vi "VD2_TRABS_Calc.vi"(8 "error in (no error)":errorcluster, 10 "Exp name":string, 11 "Control-Client in":refnum<class "Control-Client.lvclass">) -> (0 "error out":errorcluster, 3 "Control-Client out":refnum<class "Control-Client.lvclass">)   [LabVIEW 2018, in "Control-Client.lvclass"]
uses:
  Control-Client.lvclass
  Experiments/Experiment.lvclass
  Control-Client.lvclass/Control-Client.ctl
  methods/Read Group #.vi
  Experiments/Experiments_group.lvclass
panel:
  out "Item Names":string[](array[string])
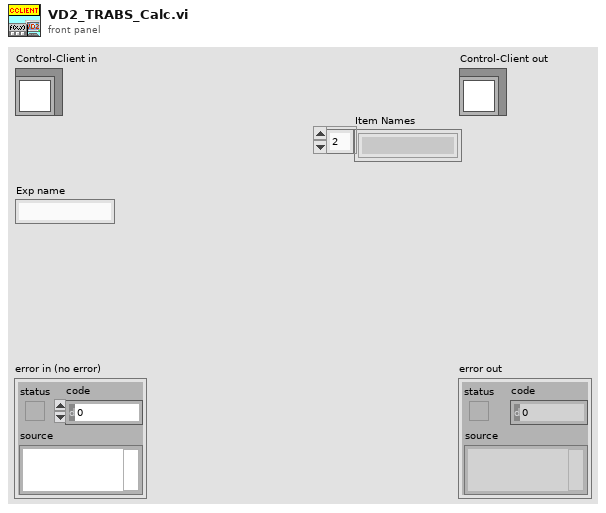
[diagram p1: front panel]
types:
  T1 = typedef "mylistbox.ctl" = i32[]
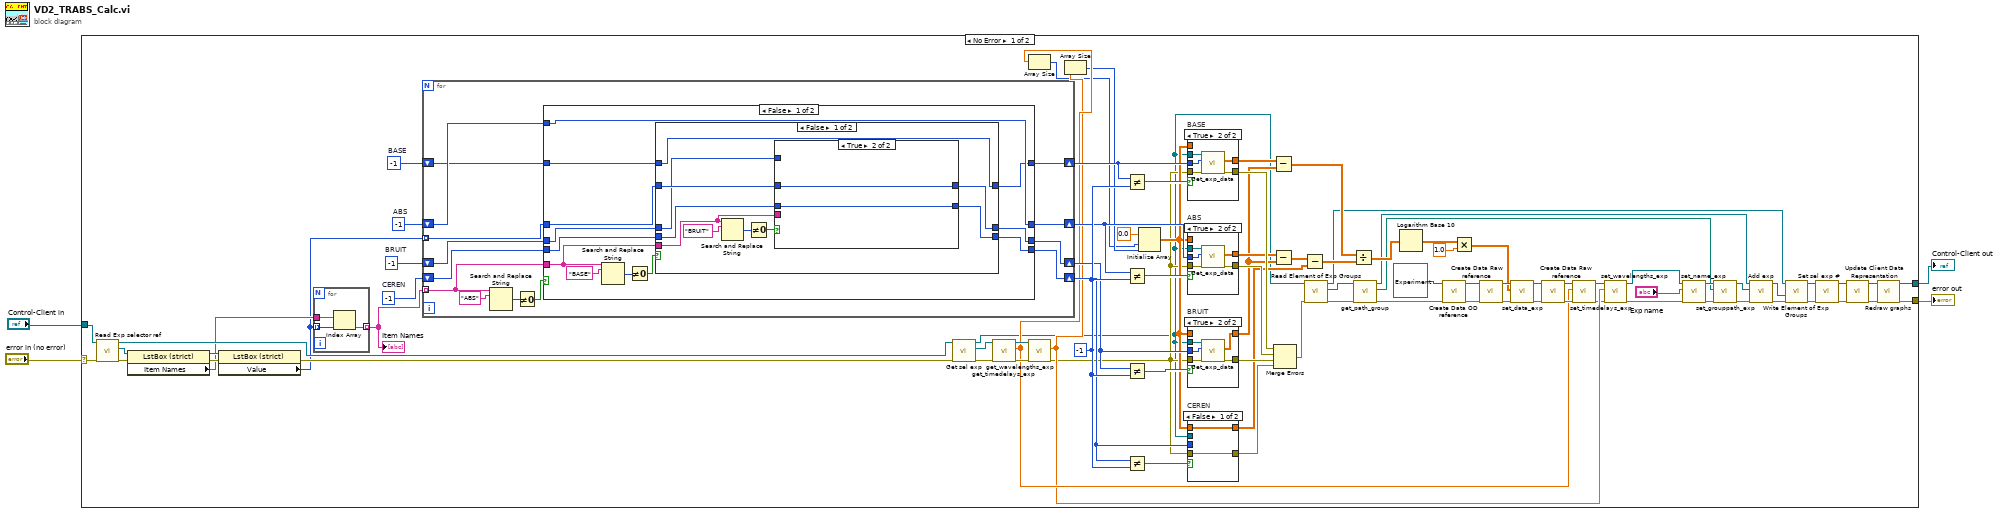
[diagram p0: block diagram]
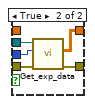
[diagram p2: hidden frame]
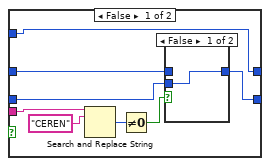
[diagram p6: hidden frame]
diagram:
  n1 = case shown="No Error" "error in (no error)" {
    selector: "error in (no error)" -> [w89 w177]
    tunnel: [w30 w177] -> w3
    tunnel: [w29 w176] -> w1
    tunnel: "Control-Client in" -> [w90 w176]
    frame No Error {
      w79 = -1 ("y")
      w85 = -1  # CEREN
      w84 = -1  # BRUIT
      w83 = -1  # BASE
      w82 = -1  # ABS
      n2 = call "Read Exp selector ref.vi"("error in (no error)"=w89, "Control-Client in"=w90) -> ("error out"=w88:errorcluster, "Exp selector ref"=w87:refnum<vi>, "Control-Client out"=w68:refnum<class "Control-Client.lvclass">)  [unwired: 7 in]
      n3 = property on="Property Node" class="LstBox (strict)"(reference=w87, error in=w88) -> (reference out=w86:refnum<vi>, error out=w19:errorcluster, "Item Names"=w17:string[])
      n4 = property class="LstBox (strict)"(reference=w86, error in=w19) -> (error out=w20:errorcluster, "Value"=w15:T1)  [unwired: 1 out]
      n5 = for {
        tunnel: w15 -> [w92] mode=indexing
        tunnel: w17 -> [w93]
        tunnel: [w91] -> w16 mode=indexing
        n6 = Index Array(array=w93, index=w92) -> (element=w91:string)
      }
      "Item Names" <- w16
      n7 = for {
        tunnel: w16 -> [w129] mode=indexing
        shift-right: [w124] -> w70
        shift-left: w85 -> [w123]
        shift-right: [w126] -> w69
        shift-left: w84 -> [w125]
        shift-right: [w128] -> w72
        shift-left: w83 -> [w127]
        shift-right: [w131] -> w71
        shift-left: w82 -> [w130]
        tunnel: w15 -> [w122] mode=indexing
        n8 = Search and Replace String(input string=w129, search string="ABS") -> (number of replacements=w133:i32)  [unwired: 6 in, 3 out]
        n9 = Not Equal To 0?(x=w133) -> (x != 0?=w132:bool)
        n10 = case shown="False" w132 {
          tunnel: [w146 w175] -> w131
          tunnel: w122 -> [w141 w175]
          tunnel: w130 -> [w146 _]
          tunnel: w129 -> [w139 _]
          tunnel: [w142 w174] -> w128
          tunnel: w127 -> [w140 w174]
          tunnel: [w138 w173] -> w126
          tunnel: w125 -> [w137 w173]
          tunnel: [w136 w172] -> w124
          tunnel: w123 -> [w135 w172]
          frame False {
            n11 = Search and Replace String(input string=w139, search string="BASE") -> (number of replacements=w144:i32)  [unwired: 6 in, 3 out]
            n12 = Not Equal To 0?(x=w144) -> (x != 0?=w143:bool)
            n13 = case shown="False" w143 {
              tunnel: [w156 w171] -> w142
              tunnel: w141 -> [w151 w171]
              tunnel: w140 -> [w156 _]
              tunnel: w139 -> [w149 _]
              tunnel: [w152 w170] -> w138
              tunnel: w137 -> [w150 w170]
              tunnel: [w148 w169] -> w136
              tunnel: w135 -> [w147 w169]
              frame False {
                n14 = Search and Replace String(input string=w149, search string="BRUIT") -> (number of replacements=w154:i32)  [unwired: 6 in, 3 out]
                n15 = Not Equal To 0?(x=w154) -> (x != 0?=w153:bool)
                n16 = case shown="True" w153 {
                  tunnel: [w164 w168] -> w152
                  tunnel: w151 -> [w158 w168]
                  tunnel: w150 -> [w164 _]
                  tunnel: w149 -> [w160 _]
                  tunnel: [w159 w167] -> w148
                  tunnel: w147 -> [w157 w167]
                  frame False {
                    n17 = Search and Replace String(input string=w160, search string="CEREN") -> (number of replacements=w162:i32)  [unwired: 6 in, 3 out]
                    n18 = Not Equal To 0?(x=w162) -> (x != 0?=w161:bool)
                    n19 = case shown="False" w161 {
                      tunnel: [w165 w166] -> w159
                      tunnel: w158 -> [_ w166]
                      tunnel: w157 -> [w165 _]
                      frame False {
                      }
                      frame True {
                      }
                    }
                  }
                  frame True {
                  }
                }
              }
              frame True {
              }
            }
          }
          frame True {
          }
        }
      }
      n20 = call "Get sel exp.vi"("error in (no error)"=w20, "Control-Client in"=w68) -> ("error out"=w66:errorcluster, "Sel experiment"=w65:refnum<class "Experiment.lvclass">, "Control-Client out"=w7:refnum<class "Control-Client.lvclass">)  [unwired: 7 in]
      n21 = call "get_timedelays_exp.vi"("error in (no error)"=w66, "Experiment.lvclass in"=w65) -> ("error out"=w67:errorcluster, "timedelays"=w27:dbl[], "Experiment.lvclass out"=w64:refnum<class "Experiment.lvclass">)  [unwired: 7 in]
      n22 = Array Size(array=w27) -> (size(s)=w5:i32)
      n23 = call "get_wavelengths_exp.vi"("error in (no error)"=w67, "Experiment.lvclass in"=w64) -> ("error out"=w18:errorcluster, "wavelengths"=w25:dbl[])  [unwired: 7 in, 1 out]
      n24 = Array Size(array=w25) -> (size(s)=w6:i32)
      n25 = Not Equal?(x=w72, y=w79) -> (x != y?=w81:bool)
      n26 = Not Equal?(x=w71, y=w79) -> (x != y?=w80:bool)
      n27 = Not Equal?(x=w69, y=w79) -> (x != y?=w78:bool)
      n28 = Not Equal?(x=w70, y=w79) -> (x != y?=w77:bool)
      n29 = Initialize Array(0.0 ("element"), w5, w6) -> (w62:dbl[][])
      n30 = case "BASE" shown="True" w81 {
        tunnel: w18 -> [w115 w121]
        tunnel: [w115 w120] -> w76
        tunnel: w7 -> [_ w119]
        tunnel: w72 -> [_ w117]
        tunnel: [w116 w118] -> w61
        tunnel: w62 -> [w116 _]
        frame False {
        }
        frame True {
          n31 = call "Get_exp_data.vi"("error in (no error)"=w121, "index"=w117, "Control-Client in"=w119) -> ("error out"=w120:errorcluster, "Data"=w118:sgl[][])  [unwired: 6 in, 1 out]
        }
      }
      n32 = case "ABS" shown="True" w80 {
        tunnel: w18 -> [w108 w114]
        tunnel: [w108 w113] -> w75
        tunnel: w7 -> [_ w112]
        tunnel: w71 -> [_ w110]
        tunnel: [w109 w111] -> w60
        tunnel: w62 -> [w109 _]
        frame False {
        }
        frame True {
          n33 = call "Get_exp_data.vi"("error in (no error)"=w114, "index"=w110, "Control-Client in"=w112) -> ("error out"=w113:errorcluster, "Data"=w111:sgl[][])  [unwired: 6 in, 1 out]
        }
      }
      n34 = case "BRUIT" shown="True" w78 {
        tunnel: w18 -> [w101 w107]
        tunnel: [w101 w106] -> w74
        tunnel: w7 -> [_ w105]
        tunnel: w69 -> [_ w103]
        tunnel: [w102 w104] -> w59
        tunnel: w62 -> [w102 _]
        frame False {
        }
        frame True {
          n35 = call "Get_exp_data.vi"("error in (no error)"=w107, "index"=w103, "Control-Client in"=w105) -> ("error out"=w106:errorcluster, "Data"=w104:sgl[][])  [unwired: 6 in, 1 out]
        }
      }
      n36 = case "CEREN" shown="False" w77 {
        tunnel: w18 -> [w95 w100]
        tunnel: [w95 w99] -> w73
        tunnel: w7 -> [_ w98]
        tunnel: w70 -> [_ w96]
        tunnel: [w94 w97] -> w57
        tunnel: w62 -> [w94 _]
        frame False {
        }
        frame True {
          n37 = call "Get_exp_data.vi"("error in (no error)"=w100, "index"=w96, "Control-Client in"=w98) -> ("error out"=w99:errorcluster, "Data"=w97:sgl[][])  [unwired: 6 in, 1 out]
        }
      }
      n38 = Subtract(x=w61, y=w59) -> (x-y=w55:dbl[][])
      n39 = Subtract(x=w60, y=w59) -> (x-y=w58:dbl[][])
      n40 = Merge Errors(w76, w75, w74, w73) -> (w14:errorcluster)
      n41 = Subtract(x=w58, y=w57) -> (x-y=w56:dbl[][])
      n42 = call "Read Element of Exp Groups.vi"("error in (no error)"=w14, "Control-Client in"=w7) -> ("error out"=w13:errorcluster, "Experiments_group.lvclass"=w10:refnum<class "Experiments_group.lvclass">, "Control-Client out"=w8:refnum<class "Control-Client.lvclass">)  [unwired: 7 in]
      n43 = Divide(x=w55, y=w56) -> (x/y=w54:dbl[][])
      n44 = call "get_path_group.vi"("error in (no error)"=w13, "Experiments_group.lvclass in"=w10) -> ("error out"=w12:errorcluster, "Path"=w11:path, "Experiments_group.lvclass out"=w9:refnum<class "Experiments_group.lvclass">)  [unwired: 7 in]
      n45 = Logarithm Base 10(1:w54) -> (0:w53:dbl[][])
      n46 = call "Create Data OD reference.vi"("error in (no error)"=w12, "Experiment in"=refnum<class "Experiment.lvclass"> refnum ("Experiment.lvclass in")) -> ("error out"=w31:errorcluster, "Experiment out"=w34:refnum<class "Experiment.lvclass">)  [unwired: 8 in]
      n47 = Multiply(x=w53, y=1.0 ("element")) -> (x*y=w28:dbl[][])
      n48 = call "Create Data Raw reference.vi"("error in (no error)"=w31, "Experiment in"=w34) -> ("error out"=w32:errorcluster, "Experiment out"=w33:refnum<class "Experiment.lvclass">)  [unwired: 8 in]
      n49 = call "set_data_exp.vi"("error in (no error)"=w32, "Data"=w28, "Experiment.lvclass in"=w33) -> ("error out"=w36:errorcluster, "Experiment.lvclass out"=w39:refnum<class "Experiment.lvclass">)  [unwired: 7 in]
      n50 = call "Create Data Raw reference.vi"("error in (no error)"=w36, "Experiment in"=w39) -> ("error out"=w37:errorcluster, "Experiment out"=w38:refnum<class "Experiment.lvclass">)  [unwired: 8 in]
      n51 = call "set_timedelays_exp.vi"("error in (no error)"=w37, "timedelays"=w27, "Experiment.lvclass in"=w38) -> ("error out"=w24:errorcluster, "Experiment.lvclass out"=w23:refnum<class "Experiment.lvclass">)  [unwired: 7 in]
      n52 = call "set_wavelengths_exp.vi"("error in (no error)"=w24, "wavelengths"=w25, "Experiment.lvclass in"=w23) -> ("error out"=w51:errorcluster, "Experiment.lvclass out"=w50:refnum<class "Experiment.lvclass">)  [unwired: 7 in]
      n53 = call "set_name_exp.vi"("error in (no error)"=w51, "Exp name"="Exp name", "Experiment.lvclass in"=w50) -> ("error out"=w41:errorcluster, "Experiment.lvclass out"=w40:refnum<class "Experiment.lvclass">)  [unwired: 7 in]
      n54 = call "set_grouppath_exp.vi"("error in (no error)"=w41, "GroupPath"=w11, "Experiment.lvclass in"=w40) -> ("error out"=w21:errorcluster, "Experiment.lvclass out"=w22:refnum<class "Experiment.lvclass">)  [unwired: 7 in]
      n55 = call "Add exp.vi"("error in (no error)"=w21, "New exp"=w22, "Experiments_group in"=w9) -> ("error out"=w46:errorcluster, "Experiments_group out"=w49:refnum<class "Experiments_group.lvclass">)  [unwired: 7 in]
      n56 = call "Write Element of Exp Groups.vi"("error in (no error)"=w46, "Experiments_group.lvclass"=w49, "Control-Client in"=w8) -> ("error out"=w47:errorcluster, "Control-Client out"=w48:refnum<class "Control-Client.lvclass">)  [unwired: 7 in]
      n57 = call "Set sel exp #.vi"("error in (no error)"=w47, "Control-Client in"=w48) -> ("error out"=w44:errorcluster, "Control-Client out"=w45:refnum<class "Control-Client.lvclass">)  [unwired: 8 in]
      n58 = call "Update Client Data Representation.vi"("error in (no error)"=w44, "Control-Client in"=w45) -> ("error out"=w43:errorcluster, "Control-Client out"=w42:refnum<class "Control-Client.lvclass">)  [unwired: 8 in]
      n59 = call "Redraw graphs.vi"("error in (no error)"=w43, "Control-Client in"=w42) -> ("error out"=w30:errorcluster, "Control-Client out"=w29:refnum<class "Control-Client.lvclass">)  [unwired: 8 in]
    }
    frame Error {
    }
  }
  "error out" <- w3
  "Control-Client out" <- w1
